vi "Create.vi"(6 "Overwrite?":bool, 8 "error in":errorcluster, 9 "SheetName":string="Sheet1", 10 "Path":path) -> (0 "error out":errorcluster, 3 "SpreadsheetDoc":refnum<k24>)   [LabVIEW 2019, in "Open Xml.lvlib"]
uses:
  Open Xml.lvlib
  D:/git/Open-Xml-LabVIEW/Source/DocumentFormat.OpenXml.dll
  DocumentFormat.OpenXml.dll
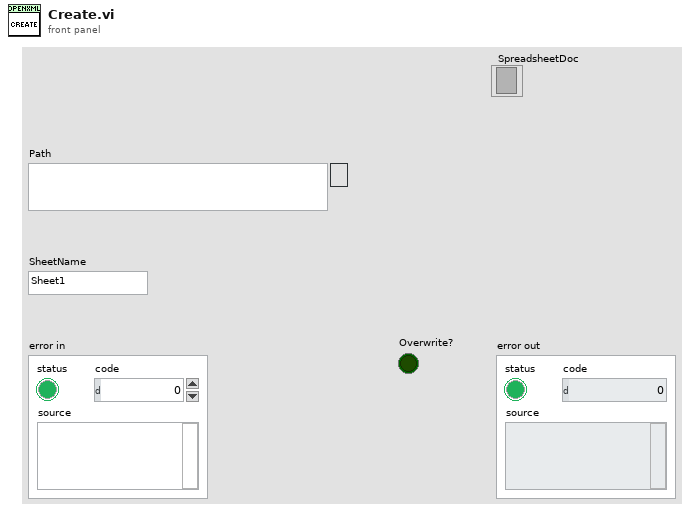
[diagram p1: front panel]
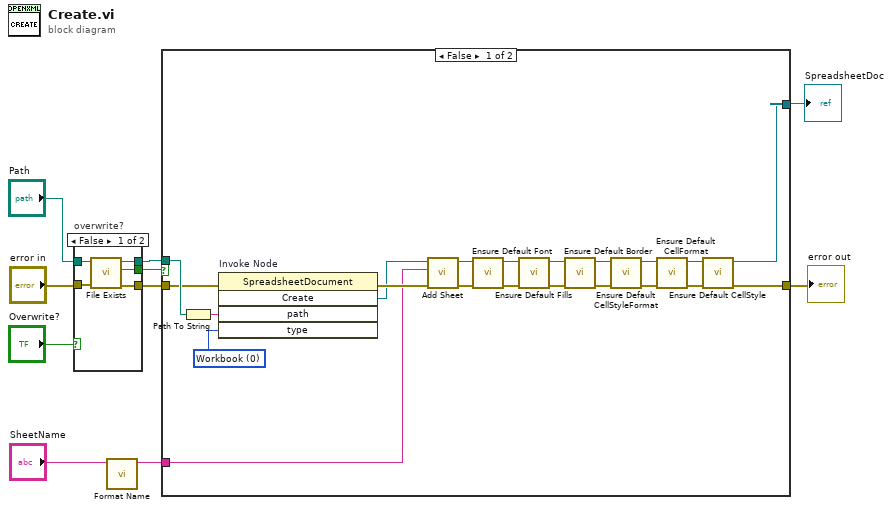
[diagram p0: block diagram]
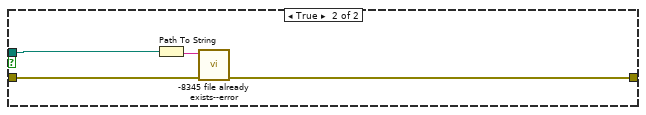
[diagram p2: hidden frame]
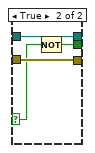
[diagram p3: hidden frame]
diagram:
  n1 = case "overwrite?" shown="False" "Overwrite?" {
    selector: "Overwrite?" -> [_ w17]
    tunnel: [w13 w16] -> w8
    tunnel: "error in" -> [w15 w19]
    tunnel: "Path" -> [w14 w18]
    tunnel: [w12 w18] -> w6
    tunnel: [w11 w19] -> w5
    frame False {
      n2 = call "File Exists.vi"("error in"=w15, "File Path"=w14) -> ("error out"=w11:errorcluster, "Exists"=w13:bool, "File Path (dup)"=w12:path)  [unwired: 7 in]
    }
    frame True {
      n3 = Not(x=w17) -> (.not. x?=w16:bool)
    }
  }
  n4 = call "Format Name.vi"("Sheet Name"="SheetName") -> ("Formatted Sheet Name"=w2:string)  [unwired: 10 in]
  n5 = case shown="False" w8 {
    tunnel: w6 -> [w40 w41]
    tunnel: w5 -> [w37 w44]
    tunnel: w2 -> [w34 _]
    tunnel: [w31 _] -> w10
    tunnel: [w30 w43] -> w3
    frame False {
      w39 = 0 items=["Workbook", "Template", "MacroEnabledWorkbook", "MacroEnabledTemplate", "AddIn"] ("Type")
      n6 = Path To String(path=w40) -> (string=w38:string)
      n7 = invoke on="Invoke Node" class="SpreadsheetDocument" method="Create"(error in=w37, "path"=w38, "type"=w39) -> (error out=w36:errorcluster, "Create"=w35:refnum<k24>)  [unwired: 2 in, 3 out]
      n8 = call "Add Sheet.vi"("error in"=w36, "Sheet Name"=w34, "SpreadsheetDoc in"=w35) -> ("error out"=w32:errorcluster, "SpreadsheetDoc out"=w33:refnum<k24>)  [unwired: 7 in]
      n9 = call "Ensure Default Font.vi"("error in"=w32, "SpreadsheetDoc in"=w33) -> ("error out"=w29:errorcluster, "SpreadsheetDoc out"=w28:refnum<k24>)  [unwired: 8 in]
      n10 = call "Ensure Default Fills.vi"("error in"=w29, "SpreadsheetDoc in"=w28) -> ("error out"=w27:errorcluster, "SpreadsheetDoc out"=w26:refnum<k24>)  [unwired: 8 in]
      n11 = call "Ensure Default Border.vi"("error in"=w27, "SpreadsheetDoc in"=w26) -> ("error out"=w25:errorcluster, "SpreadsheetDoc out"=w24:refnum<k24>)  [unwired: 8 in]
      n12 = call "Ensure Default CellStyleFormat.vi"("error in"=w25, "SpreadsheetDoc in"=w24) -> ("error out"=w23:errorcluster, "SpreadsheetDoc out"=w22:refnum<k24>)  [unwired: 8 in]
      n13 = call "Ensure Default CellFormat.vi"("error in"=w23, "SpreadsheetDoc in"=w22) -> ("error out"=w21:errorcluster, "SpreadsheetDoc out"=w20:refnum<k24>)  [unwired: 8 in]
      n14 = call "Ensure Default CellStyle.vi"("error in"=w21, "SpreadsheetDoc in"=w20) -> ("error out"=w30:errorcluster, "SpreadsheetDoc out"=w31:refnum<k24>)  [unwired: 8 in]
    }
    frame True {
      n15 = Path To String(path=w41) -> (string=w42:string)
      n16 = call "-8345 file already exists--error.vi"("error in"=w44, "Argument"=w42) -> ("error out"=w43:errorcluster)  [unwired: 9 in]
    }
  }
  "SpreadsheetDoc" <- w10
  "error out" <- w3
